vi "SSC Digital Get HRAM Trigger Settings.vi"(0 "Digital SSC in":T1[](array[typedef]), 11 "error in":errorcluster) -> (4 "Digital SSC out":T1[](array[typedef]), 6 "Per-Instrument Triggers Type":i32[](array[ring]) items=["First Failure"=2200, "Cycle Number"=2201, "Pattern Label"=2202], 8 "Per-Instrument Cycle Number Trig:Cycle Number":i64[](array[numeric]), 10 "Per-Instrument Pattern Label Trig:Pattern Label":string[](array[string]), 13 "Per-Instrument Pattern Label Trig:Cycle Offset":i64[](array[numeric]), 14 "Per-Instrument Pattern Label Trig:Vector Offset":i64[](array[numeric]), 15 "error out":errorcluster)   [LabVIEW 2019]
doc: "Uses the start label you specify to burst the pattern on the pin(s) and pin group(s) you specify."
uses:
  SSC Digital.ctl
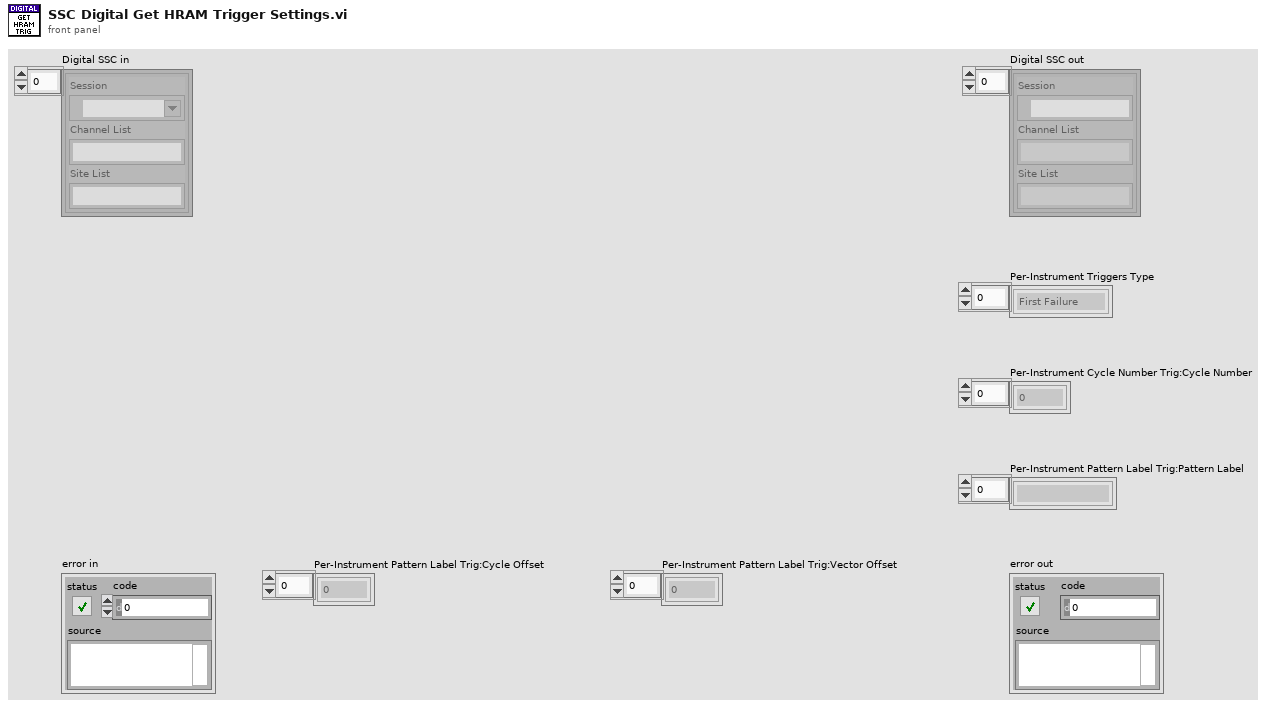
[diagram p1: front panel]
types:
  T1 = typedef "SSC Digital.ctl" = cluster{"Session":refnum<k15>, "Channel List":string, "Site List":string}
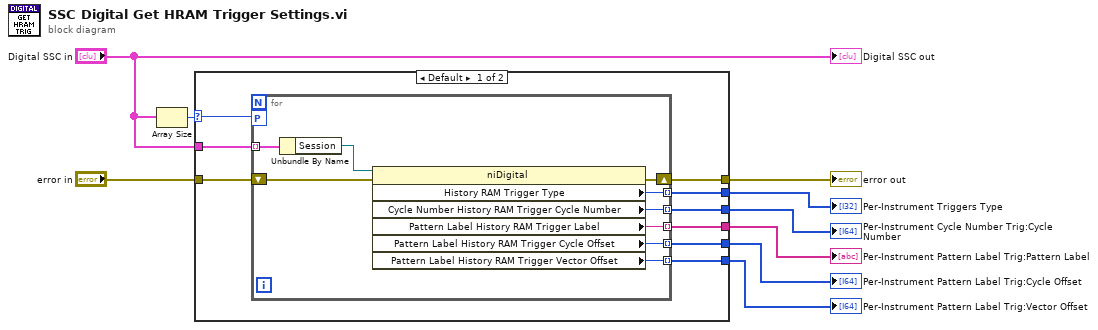
[diagram p0: block diagram]
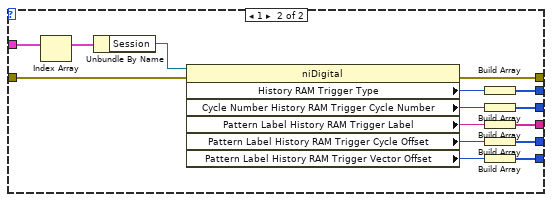
[diagram p2: hidden frame]
diagram:
  n1 = Array Size(array="Digital SSC in") -> (size(s)=w8:i32)
  n2 = case shown="Default" w8 {
    selector: w8 -> [w18 _]
    tunnel: "error in" -> [w16 w41]
    tunnel: "Digital SSC in" -> [w17 w42]
    tunnel: [w15 w40] -> w6
    tunnel: [w14 w28] -> w5
    tunnel: [w13 w29] -> w4
    tunnel: [w12 w30] -> w3
    tunnel: [w11 w31] -> w2
    tunnel: [w10 w32] -> w1
    frame Default {
      n3 = for {
        tunnel: w17 -> [w27] mode=indexing
        workers-P: w18 -> [_]
        shift-right: [w24] -> w15
        shift-left: w16 -> [w25]
        tunnel: [w23] -> w14 mode=indexing
        tunnel: [w22] -> w13 mode=indexing
        tunnel: [w21] -> w12 mode=indexing
        tunnel: [w20] -> w11 mode=indexing
        tunnel: [w19] -> w10 mode=indexing
        n4 = Unbundle By Name(w27) -> ("Session"=w26:refnum<k15>)
        n5 = property class="niDigital"(reference=w26, error in=w25) -> (error out=w24:errorcluster, "History RAM Trigger Type"=w19:i32, "Cycle Number History RAM Trigger Cycle Number"=w20:i64, "Pattern Label History RAM Trigger Label"=w21:string, "Pattern Label History RAM Trigger Cycle Offset"=w22:i64, "Pattern Label History RAM Trigger Vector Offset"=w23:i64)  [unwired: 1 out]
      }
    }
    frame 1 {
      n6 = Index Array(array=w42) -> (element=w33:T1)  [unwired: 1 in]
      n7 = Unbundle By Name(w33) -> ("Session"=w34:refnum<k15>)
      n8 = property class="niDigital"(reference=w34, error in=w41) -> (error out=w40:errorcluster, "History RAM Trigger Type"=w35:i32, "Cycle Number History RAM Trigger Cycle Number"=w36:i64, "Pattern Label History RAM Trigger Label"=w37:string, "Pattern Label History RAM Trigger Cycle Offset"=w38:i64, "Pattern Label History RAM Trigger Vector Offset"=w39:i64)  [unwired: 1 out]
      n9 = Build Array(w35) -> (w32:i32[])
      n10 = Build Array(w36) -> (w31:i64[])
      n11 = Build Array(w37) -> (w30:string[])
      n12 = Build Array(w38) -> (w29:i64[])
      n13 = Build Array(w39) -> (w28:i64[])
    }
  }
  "error out" <- w6
  "Per-Instrument Triggers Type" <- w1
  "Per-Instrument Cycle Number Trig:Cycle Number" <- w2
  "Per-Instrument Pattern Label Trig:Pattern Label" <- w3
  "Per-Instrument Pattern Label Trig:Cycle Offset" <- w4
  "Per-Instrument Pattern Label Trig:Vector Offset" <- w5
  "Digital SSC out" <- "Digital SSC in"
